vi "Z900_navX_Internal_ZeroVelocity.vi"(7 "Zero Vector":T1, 8 "error in (no error)":errorcluster, 9 "Registry":u8[](array[numeric]), 10 "Interface TypeDefs":T2 {"I2CDevRef"."Device Address" format="%.0x"}, 11 "navX Device":T8={"Interface"={"Protocol"=enum."SERIAL", "Update Rate (4Hz-60Hz)"=4, "navX Open TypeDef"=variant}, "Notify Packet"=refnum, "Loop VI Refnum"=refnum, "Ready to Close Occurrence Refnum"=refnum} {"Interface"."Update Rate (4Hz-60Hz)" min=4 max=60 step=1}) -> (0 "error out":errorcluster, 1 "Registry":u8[](array[numeric]), 2 "Interface TypeDefs":T2 {"I2CDevRef"."Device Address" format="%.0x"}, 3 "navX Device":T8={"Interface"={"Protocol"=enum."SERIAL", "Update Rate (4Hz-60Hz)"=4, "navX Open TypeDef"=variant}, "Notify Packet"=refnum, "Loop VI Refnum"=refnum, "Ready to Close Occurrence Refnum"=refnum} {"Interface"."Update Rate (4Hz-60Hz)" min=4 max=60 step=1})   [LabVIEW 2015, in "navX Library v2.lvlib"]
uses:
  navX Library v2.lvlib
  Z900_navX_DeviceTypeDef.ctl
  Z900_navX_ProtocolTypeDef.ctl
  Z900_navX_NotifyPacketTypeDef.ctl
  Z900_navX_ActionTypeDef.ctl
  Z900_navX_InterfaceTypeDef.ctl
  <vilib>/Rock Robotics/WPI/SerialPort/WPI_SerialPortRef.ctl
  <vilib>/Rock Robotics/WPI/I2C/WPI_I2CDevRef.ctl
  <vilib>/Rock Robotics/SystemInterfaces/i2clib/i2c_bus.ctl
  <vilib>/Rock Robotics/WPI/SPI/WPI_SPIDevRef.ctl
  <vilib>/Rock Robotics/SystemInterfaces/spilib/spi_bus.ctl
  Z900_navX_ZeroVectorTypeDef.ctl
  Z900_navX_DeviceRegisters.ctl
  Z900_navX_Flags_CapabilityTypeDef.ctl
  Z900_navX_IntegrationControlRegisters.ctl
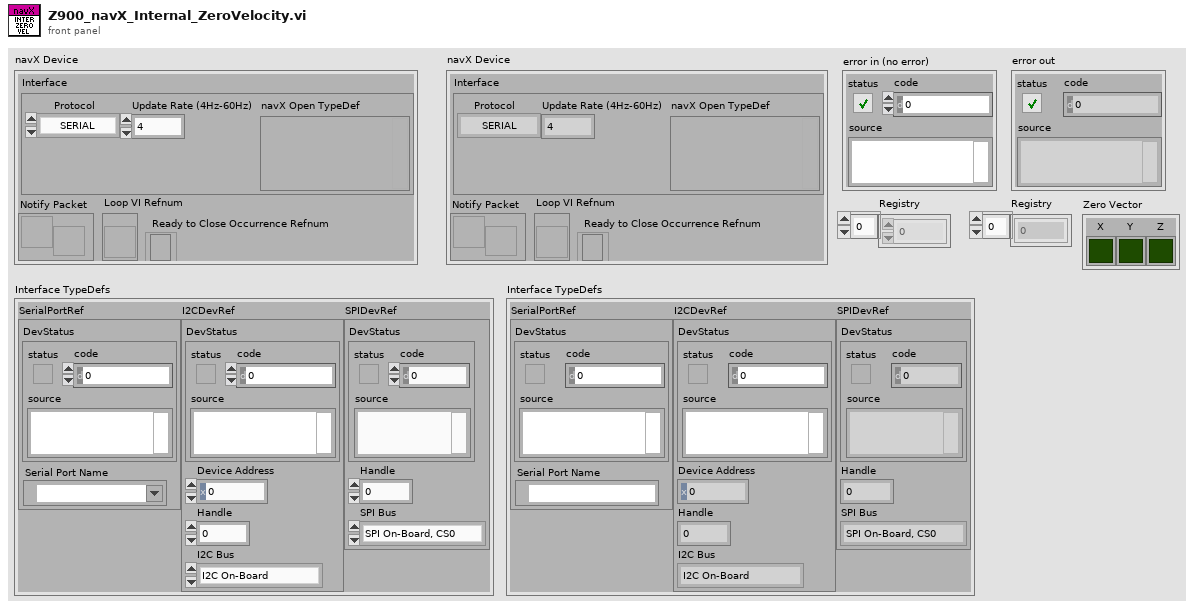
[diagram p1: front panel]
types:
  T1 = typedef "navX Library v2.lvlib/Z900_navX_ZeroVectorTypeDef.ctl" = cluster{"X":bool, "Y":bool, "Z":bool}
  T2 = typedef "navX Library v2.lvlib/Z900_navX_InterfaceTypeDef.ctl" = cluster{"SerialPortRef":T3, "I2CDevRef":T4, "SPIDevRef":T6}
  T3 = typedef "WPI_SerialPortRef.ctl" = cluster{"DevStatus":errorcluster, "Serial Port Name":refnum<visa-resource-name>}
  T4 = typedef "WPI_I2CDevRef.ctl" = cluster{"DevStatus":errorcluster, "Device Address":u8, "Handle":i32, "I2C Bus":T5}
  T5 = typedef "i2c_bus.ctl" = enum16{"I2C On-Board", "I2C MXP", "Invalid"}
  T6 = typedef "WPI_SPIDevRef.ctl" = cluster{"DevStatus":errorcluster, "Handle":i32, "SPI Bus":T7}
  T7 = typedef "spi_bus.ctl" = enum16{"SPI On-Board, CS0", "SPI On-Board, CS1", "SPI On-Board, CS2", "SPI On-Board, CS3", "SPI MXP", "Invalid"}
  T8 = typedef "navX Library v2.lvlib/Z900_navX_DeviceTypeDef.ctl" = cluster{"Interface":cluster{"Protocol":T9, "Update Rate (4Hz-60Hz)":u8, "navX Open TypeDef":variant}, "Notify Packet":refnum<notifier>, "Loop VI Refnum":refnum<vi>, "Ready to Close Occurrence Refnum":refnum<k4>}
  T9 = typedef "navX Library v2.lvlib/Z900_navX_ProtocolTypeDef.ctl" = enum16{"SERIAL", "I2C", "SPI"}
  T10 = typedef "navX Library v2.lvlib/Z900_navX_DeviceRegisters.ctl" = u8
  T11 = typedef "navX Library v2.lvlib/Z900_navX_Flags_CapabilityTypeDef.ctl" = u16
  T12 = typedef "navX Library v2.lvlib/Z900_navX_IntegrationControlRegisters.ctl" = u8
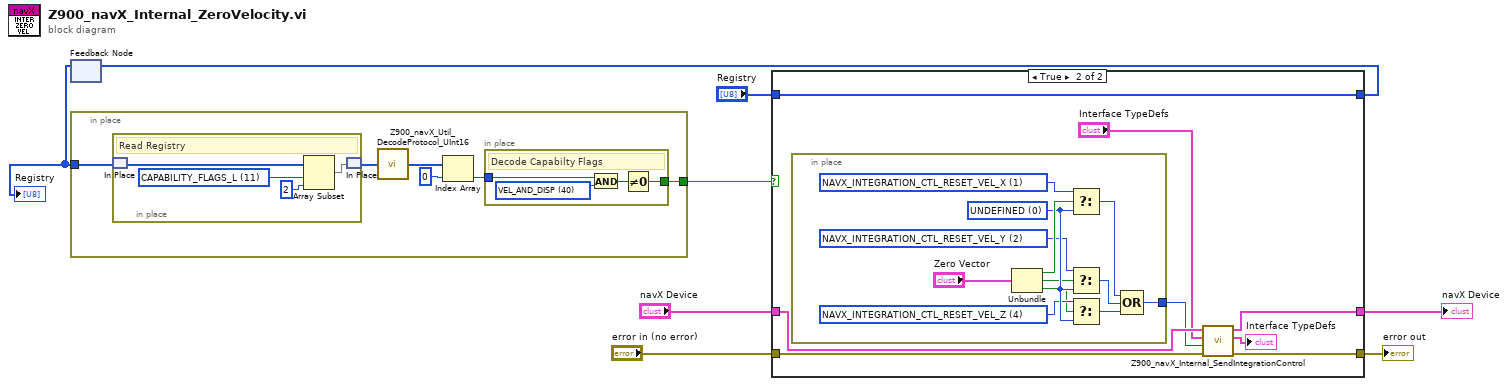
[diagram p0: block diagram]
diagram:
  n1 = feedback #1() -> (w1:u8[])  [unwired: 1 in]
  "Registry" <- w1
  n2 = in-place {
    in-place-border: w1 -> [w10]
    in-place-border: [w9] -> w8
    n3 = in-place {
      w21 = T10 11 items=["WHOAMI"=0, "HW_REV"=1, "FW_VER_MAJOR"=2, "FW_VER_MINOR"=3, "UPDATE_RATE_HZ"=4, "ACCEL_FSR_G"=5, "GYRO_FSR_DPS"=6, "OP_STATUS"=8, "CAL_STATUS"=9, "SELFTEST_STATUS"=10, "CAPABILITY_FLAGS_L"=11, "CAPABILITY_FLAGS_H"=12, "SENSOR_STATUS"=16, "TIMESTAMP"=18, "YAW"=22, "ROLL"=24, "PITCH"=26, "HEADING"=28, "FUSED_HEADING"=30, "ALTITUDE_I"=32, "ALTITUDE_D"=34, "LINERA_ACC_X"=36, "LINERA_ACC_Y"=38, "LINERA_ACC_Z"=40, "QUAT_W"=42, "QUAT_X"=44, "QUAT_Y"=46, "QUAT_Z"=48, "MPU_TEMP_C"=50, "GYRO_X"=52, "GYRO_Y"=54, "GYRO_Z"=56, "ACC_X"=58, "ACC_Y"=60, "ACC_Z"=62, "MAG_X"=64, "MAG_Y"=66, "MAG_Z"=68, "PRESSURE_I"=70, "PRESSURE_D"=72, "PRESSURE_TEMP"=74, "YAW_OFFSET"=76, "QUAT_OFFSET_W"=78, "QUAT_OFFSET_X"=80, "QUAT_OFFSET_Y"=82, "QUAT_OFFSET_Z"=84, "INTEGRATION_CONTROL"=86, "VELOCITY_X"=88, "VELOCITY_Y"=92, "VELOCITY_Z"=96, "DISPLACMENT_X"=100, "DISPLACMENT_Y"=104, "DISPLACEMENT_Z"=108] ("Device Register")
      # "Read Registry"
      n4 = in-place-match #2(w10) -> (w19:u8[])
      n5 = Array Subset(array=w19, index=w21, length=2) -> (w20:u8[])
      n6 = in-place-match #2(w20) -> (w14:u8[])
    }
    n7 = call "Z900_navX_Util_DecodeProtocol_UInt16.vi"("Little Endian"=w14) -> ("UInt16"=w13:u16[])
    n8 = Index Array(array=w13, index=0) -> (element=w12:u16)
    n9 = in-place {
      in-place-border: w12 -> [w16]
      in-place-border: [w15] -> w9
      w17 = T11 40 items=["OMNIMOUNT"=4, "OMNIMOUNT_CONFIG_MASK"=38, "VEL_AND_DISP"=40, "YAW_RESET"=80] ("Capability Flag")
      # "Decode Capabilty Flags"
      n10 = And(x=w16, y=w17) -> (x .and. y?=w18:T11)
      n11 = Not Equal To 0?(x=w18) -> (x != 0?=w15:bool)
    }
  }
  n12 = case shown="True" w8 {
    tunnel: "error in (no error)" -> [w23 w33]
    tunnel: [w23 w32] -> w3
    tunnel: "navX Device" -> [w24 w31]
    tunnel: [w24 w30] -> w6
    tunnel: "Registry" -> [w25 w29]
    tunnel: [w25 w29] -> w2
    frame False {
    }
    frame True {
      n13 = in-place {
        in-place-border: [w35] -> w28
        w43 = T12 0 items=["UNDEFINED"=0, "NAVX_INTEGRATION_CTL_RESET_VEL_X"=1, "NAVX_INTEGRATION_CTL_RESET_VEL_Y"=2, "NAVX_INTEGRATION_CTL_RESET_VEL_Z"=4, "NAVX_INTEGRATION_CTL_RESET_DISP_X"=8, "NAVX_INTEGRATION_CTL_RESET_DISP_Y"=16, "NAVX_INTEGRATION_CTL_RESET_DISP_Z"=32, "NAVX_INTEGRATION_CTL_RESET_YAW"=128] ("f")
        w42 = T12 4 items=["UNDEFINED"=0, "NAVX_INTEGRATION_CTL_RESET_VEL_X"=1, "NAVX_INTEGRATION_CTL_RESET_VEL_Y"=2, "NAVX_INTEGRATION_CTL_RESET_VEL_Z"=4, "NAVX_INTEGRATION_CTL_RESET_DISP_X"=8, "NAVX_INTEGRATION_CTL_RESET_DISP_Y"=16, "NAVX_INTEGRATION_CTL_RESET_DISP_Z"=32, "NAVX_INTEGRATION_CTL_RESET_YAW"=128] ("Integration Control Register")
        w41 = T12 2 items=["UNDEFINED"=0, "NAVX_INTEGRATION_CTL_RESET_VEL_X"=1, "NAVX_INTEGRATION_CTL_RESET_VEL_Y"=2, "NAVX_INTEGRATION_CTL_RESET_VEL_Z"=4, "NAVX_INTEGRATION_CTL_RESET_DISP_X"=8, "NAVX_INTEGRATION_CTL_RESET_DISP_Y"=16, "NAVX_INTEGRATION_CTL_RESET_DISP_Z"=32, "NAVX_INTEGRATION_CTL_RESET_YAW"=128] ("Integration Control Register")
        w44 = T12 1 items=["UNDEFINED"=0, "NAVX_INTEGRATION_CTL_RESET_VEL_X"=1, "NAVX_INTEGRATION_CTL_RESET_VEL_Y"=2, "NAVX_INTEGRATION_CTL_RESET_VEL_Z"=4, "NAVX_INTEGRATION_CTL_RESET_DISP_X"=8, "NAVX_INTEGRATION_CTL_RESET_DISP_Y"=16, "NAVX_INTEGRATION_CTL_RESET_DISP_Z"=32, "NAVX_INTEGRATION_CTL_RESET_YAW"=128] ("Integration Control Register")
        n14 = Unbundle("Zero Vector") -> ("X"=w45:bool, "Y"=w40:bool, "Z"=w39:bool)
        n15 = Select(t=w44, s=w45, f=w43) -> (s? t:f=w38:T12)
        n16 = Select(t=w41, s=w40, f=w43) -> (s? t:f=w37:T12)
        n17 = Select(t=w42, s=w39, f=w43) -> (s? t:f=w36:T12)
        n18 = Compound Arithmetic op=OR(w38, w37, w36) -> (w35:T12)
      }
      n19 = call "Z900_navX_Internal_SendIntegrationControl.vi"("error in (no error)"=w33, "Integration Control Register"=w28, "Interface TypeDefs"="Interface TypeDefs", "navX Device"=w31) -> ("error out"=w32:errorcluster, "Interface TypeDefs"=→"Interface TypeDefs":T2, "navX Device"=w30:T8)  [unwired: 5 in]
    }
  }
  "error out" <- w3
  "navX Device" <- w6
  n20 = feedback-in #1(w2) -> ()
